vi "Load Action Points.vi"(8 "Error In":errorcluster, 10 "Source":string) -> (0 "Error Out":errorcluster)   [LabVIEW 2024, in "Instrument Manager.lvclass"]
uses:
  Instrument Manager.lvclass
  Instrument Manager.lvclass/Instrument Manager.ctl
  03154150-9636-41b2-8ac1-c8a1f310a941.vi
  Config from JSON/Config from JSON.lvclass
  cb9950d8-d4aa-49c1-82d4-aba589317de2.vi
  <vilib>/Utility/Data Type/NI_Data Type.lvlib
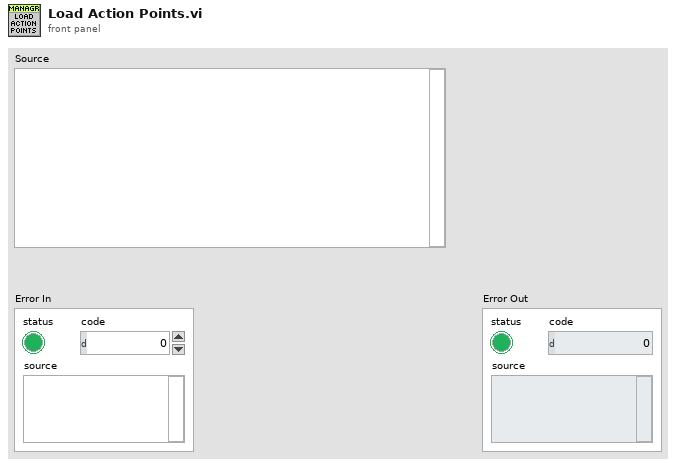
[diagram p1: front panel]
types:
  T1 = typedef "Instrument Manager.lvclass/ObjectAttributes.ctl" = cluster{"ICreate Action Point":refnum<class "ICreate Action Point.lvclass">, "IInstruments":map{string, refnum<class "IInstrument.lvclass">}, "IVirtual Instruments":map{string, refnum<class "IVirtual Instrument.lvclass">}, "Instrument Configurations":map{string, refnum<class "Config from JSON.lvclass">}, "Virtual Instrument Configurations":map{string, refnum<class "Config from JSON.lvclass">}, "Action Point Configurations":map{string, refnum<class "Config from JSON.lvclass">}, "Action Points":map{string, refnum<class "Action Point.lvclass">}}
  T2 = map{string, refnum<class "Config from JSON.lvclass">}
  T3 = typedef "NI_Data Type.lvlib/Data Type.ctl" = enum8{"Invalid Type", "Void", "I8", "I16", "I32", "I64", "U8", "U16", "U32", "U64", "Single Float", "Double Float", "Extended Float", "Single Complex", "Double Complex", "Extended Complex", "Enum U8", "Enum U16", "Enum U32", "Enum U64", "Single Float With Unit", "Double Float With Unit", "Extended Float With Unit", "Single Complex with Unit", "Double Complex with Unit", "Extended Complex with Unit", "Boolean", "String", "Path", "Picture", "Tag", "Array", "Cluster", "Variant", "LV Variant", "Waveform", "Timestamp", "Digital Waveform", "Digital Data", "ExpressData", "Refnum", "External Data", "VI", "Poly VI", "LabVIEW Class Instance", "Fixed Point", "Set Collection", "Map Collection"}
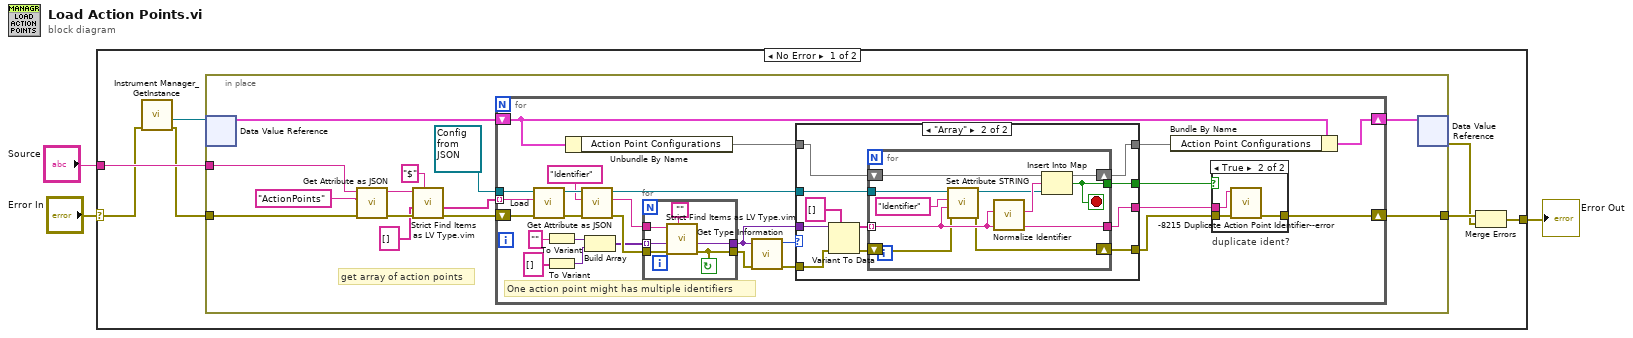
[diagram p0: block diagram]
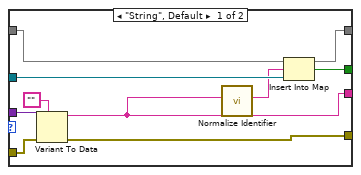
[diagram p2: hidden frame]
diagram:
  n1 = case shown="No Error" "Error In" {
    selector: "Error In" -> [w9 w91]
    tunnel: [w5 w91] -> w3
    tunnel: "Source" -> [w10 _]
    frame No Error {
      n2 = call "Instrument Manager_GetInstance.vi"("Error In"=w9) -> ("Error Out"=w8:errorcluster, "DVRRefOut"=w6:refnum<data-value>)  [unwired: 6 in, 3 out]
      n3 = in-place {
        in-place-border: w10 -> [w18]
        in-place-border: w8 -> [w23]
        in-place-border: [w20] -> w7
        # "get array of action points"
        n4 = in-place-dvr #1(w6) -> (w21:T1)  [unwired: 1 out]
        n5 = call "Get Attribute as JSON.vi"("error in"=w23, "Attribute"="ActionPoints", "Source"=w18) -> ("error out"=w22:errorcluster, "<JSON>"=w17:string)  [unwired: 7 in]
        n6 = call "Strict Find Items as LV Type.vim"("$Path or Item Name"="$", "error in"=w22, "Data Type and Default Value"=string[] [], "<JSON>"=w17) -> ("error out"=w14:errorcluster, "Data out"=w13:string[])  [unwired: 5 in, 1 out]
        n7 = for {
          shift-right: [w47] -> w20
          shift-left: w14 -> [w49]
          tunnel: w13 -> [w44] mode=indexing
          shift-right: [w45] -> w19
          shift-left: w21 -> [w46]
          tunnel: refnum<class "Config from JSON.lvclass"> refnum ("Config From JSON in") -> [w43]
          # "One action point might has multiple identifiers"
          n8 = call-dynamic "Load.vi"("error in"=w49, "Source"=w44, "Config From JSON in"=w43) -> ("error out"=w48:errorcluster, "Config From JSON out"=w42:refnum<class "Config from JSON.lvclass">)  [unwired: 7 in]
          n9 = To Variant(anything="") -> (Variant=w39:variant)
          n10 = To Variant(anything=string[] []) -> (Variant=w24:variant)
          n11 = Unbundle By Name(w46) -> ("Action Point Configurations"=w32:T2)
          n12 = call-dynamic "Get Attribute as JSON.vi"("error in"=w48, "Attribute"="Identifier" ("$Path or Item Name"), "Config from JSON in"=w42) -> ("error out"=w40:errorcluster, "<JSON>"=w37:string, "Config from JSON out"=w29:refnum<class "Config from JSON.lvclass">)  [unwired: 6 in]
          n13 = Build Array(w39, w24) -> (w38:variant[])
          n14 = for {
            tunnel: w40 -> [w86]
            tunnel: w38 -> [w84] mode=indexing
            tunnel: w37 -> [w83]
            tunnel: [w82] -> w36
            tunnel: [w81] -> w33
            stop <- w82 continue-if-true
            n15 = call "Strict Find Items as LV Type.vim"("$Path or Item Name"="", "error in"=w86, "Data Type and Default Value"=w84, "<JSON>"=w83) -> ("error out"=w82:errorcluster, "Data out"=w81:variant)  [unwired: 5 in, 1 out]
          }
          n16 = call <vilib>:"Get Type Information.vi"("error in (no error)"=w36, "variant"=w33) -> ("error out"=w34:errorcluster, "type"=w35:T3)  [unwired: 5 in, 3 out]
          n17 = case shown="\"Array\"" w35 {
            tunnel: w34 -> [w58 w68]
            tunnel: w33 -> [w59 w69]
            tunnel: w32 -> [w54 w66]
            tunnel: [w51 w62] -> w31
            tunnel: [w56 w63] -> w30
            tunnel: w29 -> [w55 w67]
            tunnel: [w53 w65] -> w28
            tunnel: [w52 w60] -> w27
            frame "String", Default {
              n18 = Variant To Data(error in=w58, type="", Variant=w59) -> (data=w51:string, error out=w52:errorcluster)
              n19 = call "Normalize Identifier.vi"("Identifier"=w51) -> ("Normalized Identifier"=w50:string)  [unwired: 10 in]
              n20 = Insert Into Map(map in=w54, key=w50, value=w55) -> (map out=w53:T2, key already included?=w56:bool)  [unwired: 1 out]
            }
            frame "Array" {
              n21 = Variant To Data(error in=w68, type=string[] [], Variant=w69) -> (data=w64:string[], error out=w61:errorcluster)
              n22 = for {
                tunnel: w67 -> [w80]
                shift-right: [w78] -> w65
                shift-left: w66 -> [w79]
                tunnel: w64 -> [w73] mode=indexing
                tunnel: [w77] -> w63
                tunnel: [w73] -> w62
                shift-right: [w71] -> w60
                shift-left: w61 -> [w72]
                stop <- w77 stop-if-true
                n23 = call-dynamic "Set Attribute STRING.vi"("error in"=w72, "Value"=w73, "Path"="Identifier", "Config from JSON in"=w80) -> ("error out"=w71:errorcluster, "Config from JSON out"=w75:refnum<class "Config from JSON.lvclass">)  [unwired: 6 in]
                n24 = call "Normalize Identifier.vi"("Identifier"=w73) -> ("Normalized Identifier"=w76:string)  [unwired: 10 in]
                n25 = Insert Into Map(map in=w79, key=w76, value=w75) -> (map out=w78:T2, key already included?=w77:bool)  [unwired: 1 out]
              }
            }
          }
          n26 = Bundle By Name(cluster=w46, "Action Point Configurations"=w28) -> (w45:T1)
          n27 = case "duplicate ident?" shown="True" w30 {
            tunnel: w27 -> [w87 w90]
            tunnel: [w87 w89] -> w47
            tunnel: w31 -> [_ w88]
            frame False {
            }
            frame True {
              n28 = call "-8215 Duplicate Action Point Identifier--error.vi"("error in"=w90, "Action Point Identifier"=w88) -> ("error out"=w89:errorcluster)  [unwired: 9 in]
            }
          }
        }
        n29 = in-place-dvr #1(w19) -> (w4:errorcluster)  [unwired: 1 out]
      }
      n30 = Merge Errors(w7, w4) -> (w5:errorcluster)
    }
    frame Error {
    }
  }
  "Error Out" <- w3
